vi "Lab4_Ex2.vi"() -> ()   [LabVIEW 2019]
uses:
  <vilib>/Utility/file.llb/Read Delimited Spreadsheet (string).vi
panel:
  in  "OK Button":bool
  in  "file path (dialog if empty)":path
  out "File Contents":string
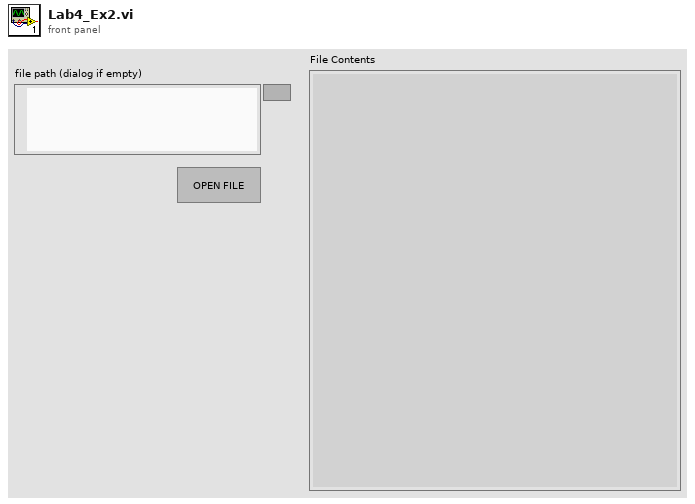
[diagram p1: front panel]
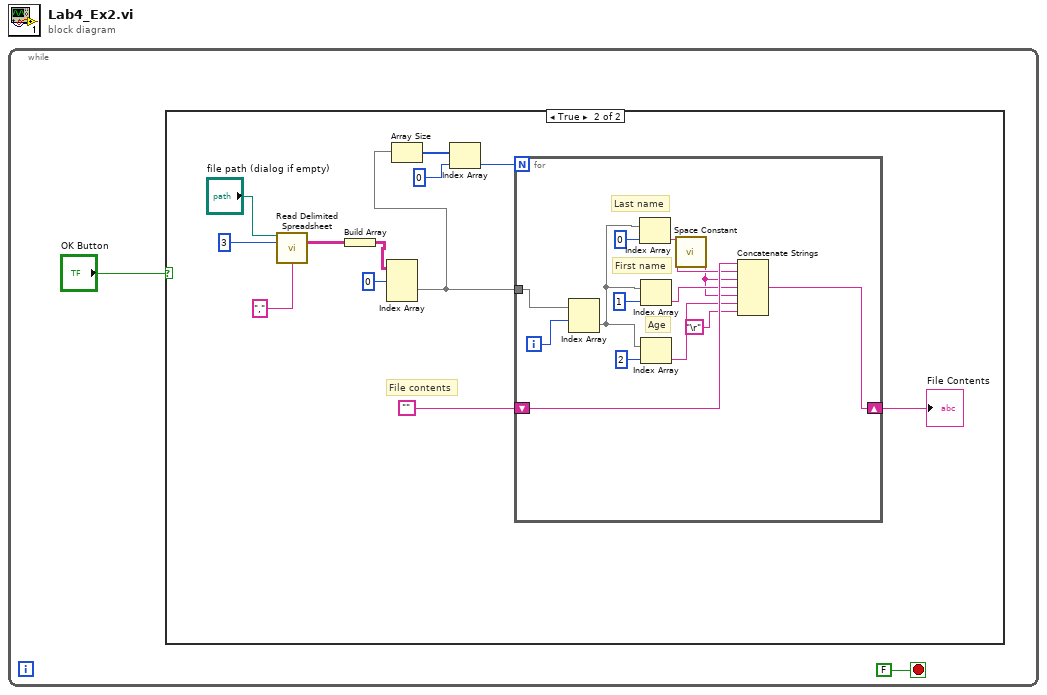
[diagram p0: block diagram]
diagram:
  n1 = while {
    stop <- FALSE stop-if-true
    n2 = case shown="True" "OK Button" {
      frame False {
      }
      frame True {
        # "File contents"
        n3 = call-poly <vilib>:"Read Delimited Spreadsheet.vi"("file path (dialog if empty)"="file path (dialog if empty)", "number of rows (all:-1)"=3, "delimiter (\\t)"=",") -> ("all rows"=w14:string[][])  [unwired: 7 in, 5 out]
        n4 = Build Array(w14) -> (w5:string[][][])
        n5 = Index Array(array=w5, index (dim 0)=0) -> (element=w3:string[][])  [unwired: 2 in]
        n6 = Array Size(array=w3) -> (size(s)=w7:i32[])
        n7 = Index Array(array=w7, index=0) -> (element=w6:i32)
        n8 = for {
          N: w6 -> [_]
          shift-right: [w21] -> w8
          shift-left: "" -> [w27]
          tunnel: w3 -> [w23]
          i -> [w20]
          # "Age"
          # "First name"
          # "Last name"
          n9 = Index Array(array=w23, index (row)=w20) -> (element=w22:string[])  [unwired: 1 in]
          n10 = Index Array(array=w22, index=0) -> (element=w19:string)
          n11 = Index Array(array=w22, index=1) -> (element=w16:string)
          n12 = Index Array(array=w22, index=2) -> (element=w18:string)
          n13 = call <vilib>:"Space Constant.vi"() -> ("String"=w15:string)
          n14 = Concatenate Strings(w27, w19, w15, w16, w15, w18, "\r") -> (w21:string)
        }
        "File Contents" <- w8
      }
    }
  }
